vi "keydown.vi"() -> ()   [LabVIEW 2015]
doc: "This VI shows how to use the Key Down Event in the LabVIEW event structure to determine keyboard selections, including modifiers, made by the user. When run, the VI waits on keyboard input from the user. The Key Down Event will detect the key that is depressed, as well as if it is modified by the Alt, Ctrl, or Shift key.\n\nIn this example, if the character pressed is an ASCII character, indicated by the value of the VKey output, the value is converted into a string, and displayed. To illustrate the use of the modifier keys, the user can press Ctrl+Shift+Q to stop the VI.\n\nThis VI also illustrates the LabVIEW's ability to discard Events. If the Discard Event Boolean is on, then LabVIEW will still detect Key Down Events, but it will not process them. So if Discard Event is on, the user cannot type text into a text box; the keystrokes will be received, but not processed by the user interface.\n\nIt is important to note that the Discard Event boolean does not prevent the execution of code based on user input. It only applies to the user interface. If Discard Event is on, the Escape key, which has been assigned via Key Navigation to the Stop button (right click... Advanced --> Key Navigation) will be detected, but the user interface will ignore it. However, the code that checks the key value still executes, and will stop the VI."
uses:
  <vilib>/event_ctls.llb/eventvkey.ctl
panel:
  in  "Discard Event":bool
  in  "Test Area":string="Type Text Here"
  out "Character Pressed (if ASCII)":string
  out "VKey":T1=enum."Enter"
  out "Value of Character Pressed":i16
  out "Modifier(s)":T2
  in  "Stop":bool
  # "For an explanation of the features that this VI demonstrates, please see the VI Documentation (Ctrl +I)."
  # "(Text will not appear if \"Ignore Event\" is on)"
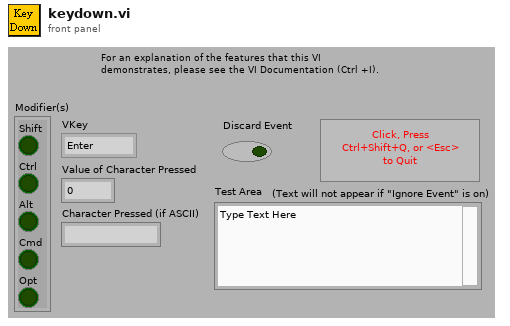
[diagram p1: front panel]
types:
  T1 = typedef "eventvkey.ctl" = enum16{"ASCII", "Enter", "Return", "Shift", "Ctrl", "Alt", "Cmd", "Opt", "Caps", "NumLock", "Clear", "Break", "Up", "Down", "Left", "Right", "Insert", "Delete", "Home", "End", "PageUp", "PageDown", "Escape", "Help", "Pause", "ScrollLock", "F1", "F2", "F3", "F4", "F5", "F6", "F7", "F8", "F9", "F10", "F11", "F12", "F13", "F14", "F15", "F16", "F17", "F18", "F19", "F20", "F21", "F22", "F23", "F24", "Play", "VolumeUp", "VolumeDown", "Mute", "Two Byte Char"}
  T2 = cluster{"Shift":bool, "Ctrl":bool, "Alt":bool, "Cmd":bool, "Opt":bool}
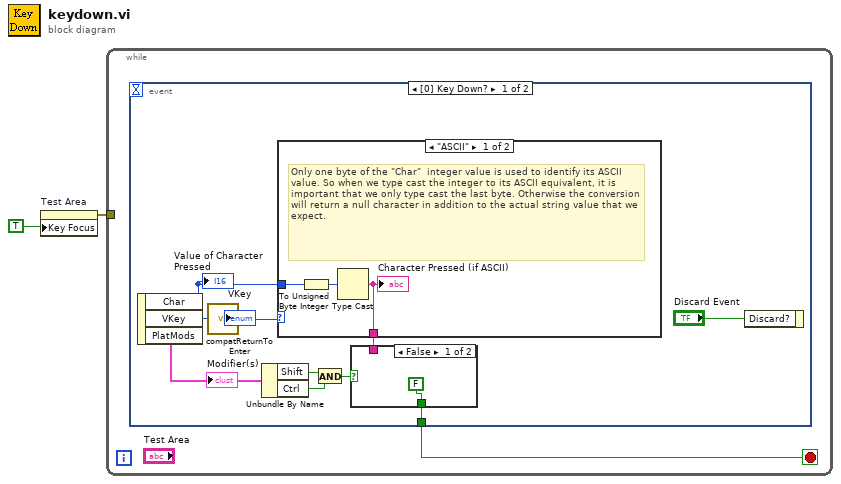
[diagram p0: block diagram]
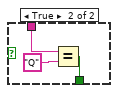
[diagram p2: hidden frame]
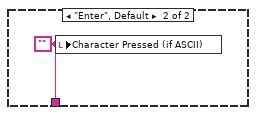
[diagram p3: hidden frame]
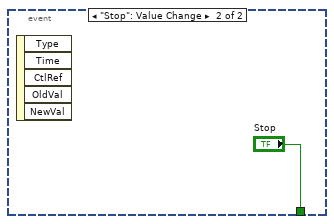
[diagram p4: hidden frame]
diagram:
  n1 = property on="Test Area" class="Str"("Key Focus"=TRUE) -> (error out=w2:errorcluster)  [unwired: 2 in, 1 out]
  n2 = while {
    tunnel: w2 -> [_]
    stop <- w3 stop-if-true
    n3 = event shown="[0] Key Down?" {
      selector: _ -> [_ _]
      dyn-events: _ -> [_ _]
      timeout: _ -> [_ _]
      tunnel: [w6 "Stop"] -> w3
      event Key Down? {
        n4 = event-data() -> ("Char"=w12:i16, "VKey"=w4:T1, "PlatMods"=w11:T2)  [unwired: 1 in]
        "Modifier(s)" <- w11
        "Value of Character Pressed" <- w12
        n5 = call <vilib>:"compatReturnToEnter.vi"("VKey"=w4) -> ("VKey"=w13:T1)
        "VKey" <- w13
        n6 = Unbundle By Name(w11) -> ("Shift"=w9:bool, "Ctrl"=w8:bool)
        n7 = case shown="\"ASCII\"" w13 {
          tunnel: w12 -> [w19 _]
          tunnel: [w18 w21] -> w7
          frame "ASCII" {
            # "Only one byte of the \"Char\"  integer value is used to identify its ASCII value. So when we type cast the integer to its ASCII equivalent, it is important that we only type cast the last byte. Otherwise the conversion will return a null character in addition to the actual string value that we expect."
            n8 = To Unsigned Byte Integer(number=w19) -> (unsigned 8bit integer=w20:u8)
            n9 = Type Cast(x=w20) -> (*(type *) &x=w18:string)  [unwired: 1 in]
            "Character Pressed (if ASCII)" <- w18
          }
          frame "Enter", Default {
            w21 = ""
            n10 = local write "Character Pressed (if ASCII)"(w21) -> ()
          }
        }
        n11 = And(x=w9, y=w8) -> (x .and. y?=w10:bool)
        n12 = case shown="False" w10 {
          tunnel: w7 -> [_ w15]
          tunnel: [FALSE w16] -> w6
          frame False {
          }
          frame True {
            n13 = Equal?(x=w15, y="Q") -> (x = y?=w16:bool)
          }
        }
        n14 = event-data("Discard?"="Discard Event") -> ()  [unwired: 1 in, 1 out]
      }
      event "Stop": Value Change {
        n15 = event-data() -> ()  [unwired: 1 in, 5 out]
      }
    }
  }
